vi "test--find free labels on fp.vi"() -> ()   [LabVIEW 2021]
uses:
  <vilib>/Utility/miscctls.llb/LVPositionTypeDef.ctl
  <vilib>/Utility/traverseref.llb/TRef TravTarget.ctl
  <vilib>/Utility/traverseref.llb/VI Scripting - Traverse.lvlib
panel:
  out "error out":errorcluster
  out "Array 2":u32[](array[colorbox])
  out "Array":T1[](array[typedef])
  out "# of Refs":i32
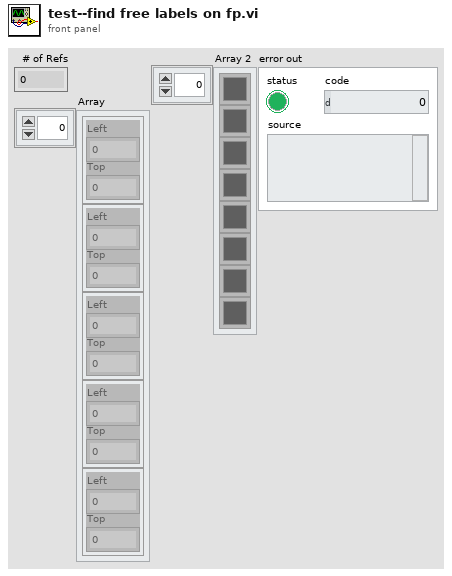
[diagram p1: front panel]
types:
  T1 = typedef "LVPositionTypeDef.ctl" = cluster{"Left":i32, "Top":i32}
  T2 = typedef "TRef TravTarget.ctl" = enum16{"FP", "BD", "Other"}
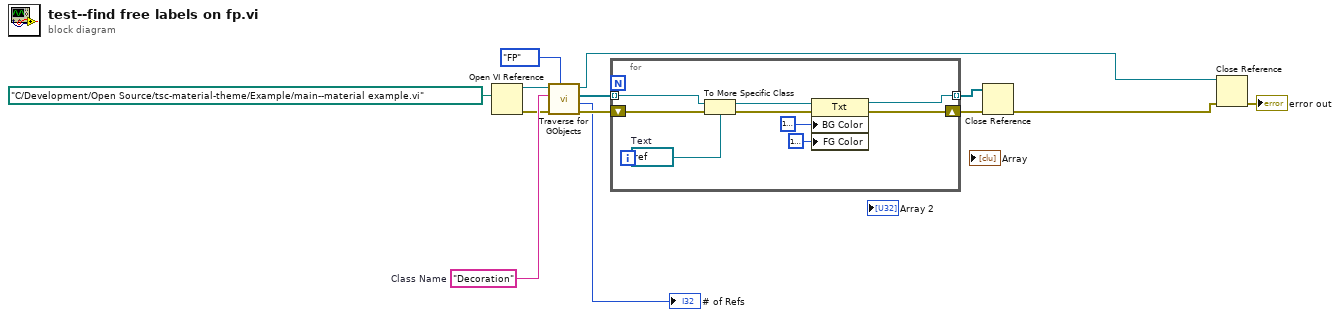
[diagram p0: block diagram]
diagram:
  w13 = "Decoration"  # Class Name
  n1 = Open VI Reference(vi path=path "C:/Development/Open Source/tsc-material-theme/Example/main--material example.vi") -> (vi reference=w9:refnum<vi>, error out=w8:errorcluster)  [unwired: 5 in]
  n2 = call <vilib>:"Traverse for GObjects.vi"("Traverse Target"=TRef_TravTarget."FP", "error in (no error)"=w8, "Class Name"=w13, "VI Refnum"=w9) -> ("error out"=w12:errorcluster, "# of Refs"=→"# of Refs":i32, "References"=w11:refnum<vi>[], "dup VI Refnum"=w2:refnum<vi>)  [unwired: 4 in]
  n3 = for {
    tunnel: w11 -> [w19] mode=indexing
    shift-right: [w18] -> w6
    shift-left: w12 -> [w22]
    tunnel: [w16] -> w3 mode=indexing
    w20 = refnum<vi> refnum  # Text
    n4 = To More Specific Class(target class=w20, reference=w19, error in=w22) -> (specific class reference=w17:refnum<vi>, error out=w21:errorcluster)
    n5 = property class="Txt"(reference=w17, error in=w21, "BG Color"=u32 16777216 ("Colors:FG Color"), "FG Color"=u32 16777216 ("Colors:FG Color")) -> (reference out=w16:refnum<vi>, error out=w18:errorcluster)
  }
  n6 = Close Reference(reference=w3, error in (no error)=w6) -> (error out=w4:errorcluster)
  n7 = Close Reference(reference=w2, error in (no error)=w4) -> (error out=→"error out":errorcluster)
